vi "JUnit Full.vi"() -> ()   [LabVIEW 2013]
doc: "This example illustrates how to create a complete JUnit XML report."
uses:
  JUnit XML/Test Suites/Test Suites.lvclass
  <vilib>/xml/Close Reference(Node).vi
  <vilib>/xml/NI_XML.lvlib
  <resource>/objmgr/DOMUserDefRef.rc
  JUnit XML/Test Case/Test Case.lvclass
  JUnit XML/Test Suite/Test Suite.lvclass
  JUnit XML/Property/Property.lvclass
panel:
  out "XML":string
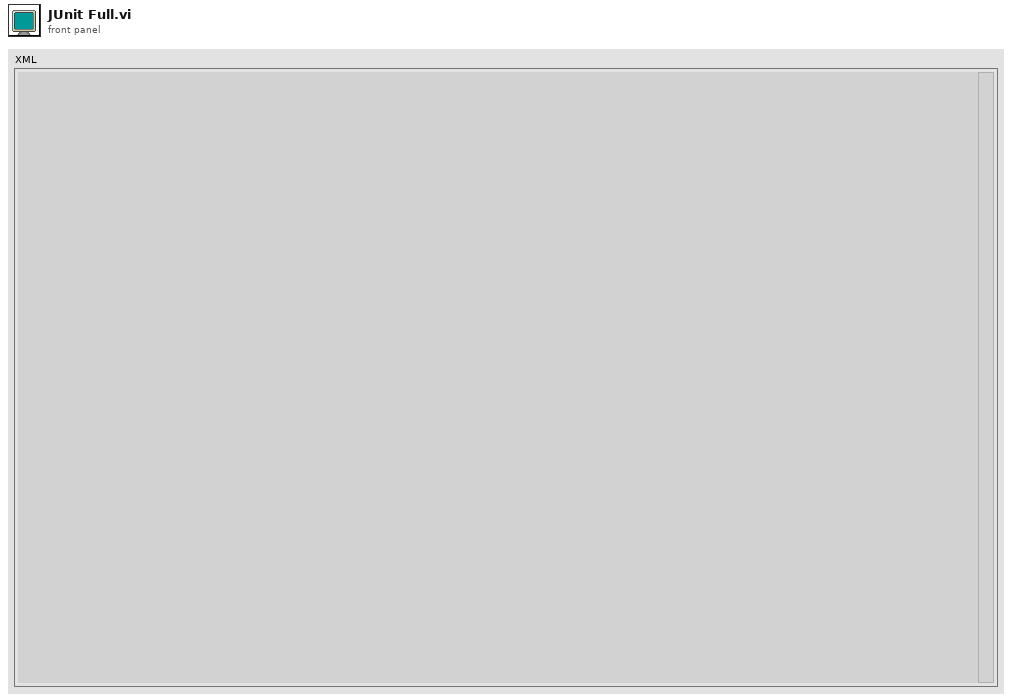
[diagram p1: front panel]
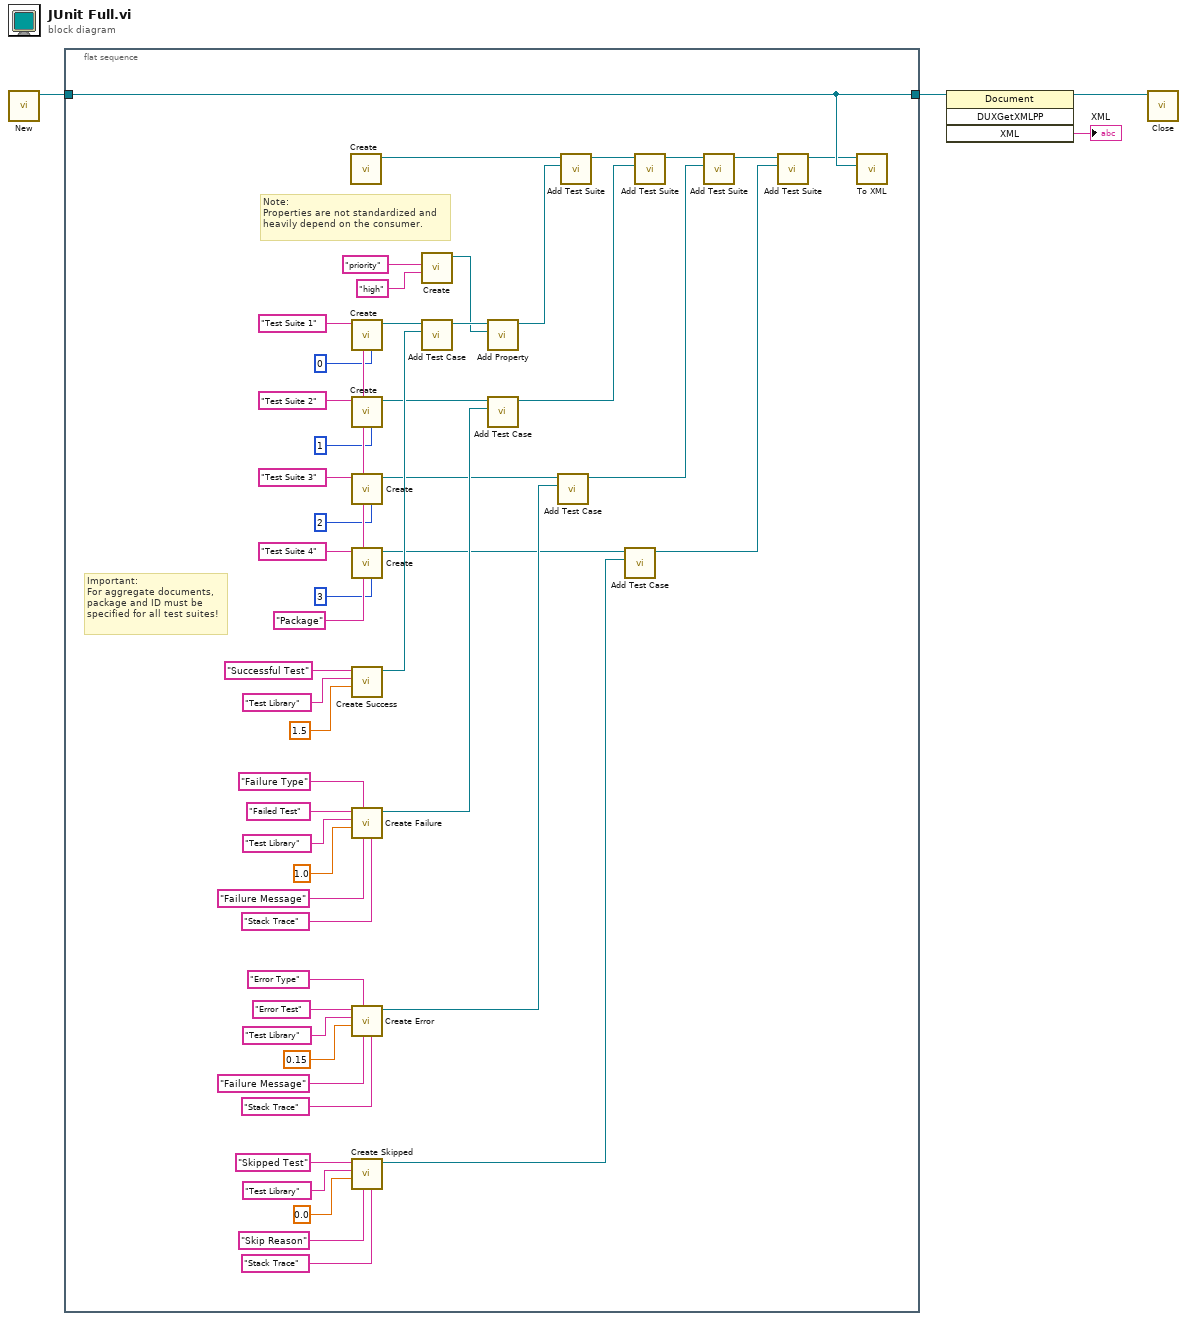
[diagram p0: block diagram]
diagram:
  n1 = call <vilib>:"New.vi"() -> ("DOM document out"=w4:refnum<k20>)  [unwired: 8 in, 1 out]
  n2 = flat-sequence {
    tunnel: w4 -> [w49]
    tunnel: [w49] -> w2
    frame #0 {
      w14 = "Package" ("Package (\"\" = undefined)")
      # "Note:\nProperties are not standardized and\nheavily depend on the consumer."
      # "Important:\nFor aggregate documents,\npackage and ID must be\nspecified for all test suites!"
      n3 = call "Create.vi"() -> ("Test Suites"=w28:refnum<class "Test Suites.lvclass">)  [unwired: 10 in, 1 out]
      n4 = call "Create.vi"("Id (-1 = undefined)"=0, "Package (\"\" = undefined)"=w14, "Name"="Test Suite 1") -> ("Test Suite"=w51:refnum<class "Test Suite.lvclass">)  [unwired: 7 in, 1 out]
      n5 = call "Create.vi"("Id (-1 = undefined)"=1, "Package (\"\" = undefined)"=w14, "Name"="Test Suite 2") -> ("Test Suite"=w24:refnum<class "Test Suite.lvclass">)  [unwired: 7 in, 1 out]
      n6 = call "Create.vi"("Id (-1 = undefined)"=2, "Package (\"\" = undefined)"=w14, "Name"="Test Suite 3") -> ("Test Suite"=w23:refnum<class "Test Suite.lvclass">)  [unwired: 7 in, 1 out]
      n7 = call "Create.vi"("Id (-1 = undefined)"=3, "Package (\"\" = undefined)"=w14, "Name"="Test Suite 4") -> ("Test Suite"=w22:refnum<class "Test Suite.lvclass">)  [unwired: 7 in, 1 out]
      n8 = call "Create Success.vi"("Time"=1.5, "Classname"="Test Library", "Name"="Successful Test") -> ("Test Case"=w50:refnum<class "Test Case.lvclass">)  [unwired: 7 in, 1 out]
      n9 = call "Create Failure.vi"("Stack Trace"="Stack Trace", "Message"="Failure Message", "Type"="Failure Type", "Time"=1.0, "Classname"="Test Library", "Name"="Failed Test") -> ("Test Case"=w42:refnum<class "Test Case.lvclass">)  [unwired: 4 in, 1 out]
      n10 = call "Create Error.vi"("Stack Trace"="Stack Trace", "Message"="Failure Message", "Type"="Error Type", "Time"=0.15, "Classname"="Test Library", "Name"="Error Test") -> ("Test Case"=w35:refnum<class "Test Case.lvclass">)  [unwired: 4 in, 1 out]
      n11 = call "Create Skipped.vi"("Stack Trace"="Stack Trace", "Message"="Skip Reason", "Time"=0.0, "Classname"="Test Library", "Name"="Skipped Test") -> ("Test Case"=w29:refnum<class "Test Case.lvclass">)  [unwired: 5 in, 1 out]
      n12 = call "Create.vi"("Value"="high", "Name"="priority") -> ("Property"=w7:refnum<class "Property.lvclass">)  [unwired: 8 in, 1 out]
      n13 = call "Add Test Case.vi"("Test Case"=w50, "Test Suite in"=w51) -> ("Test Suite out"=w9:refnum<class "Test Suite.lvclass">)  [unwired: 8 in, 1 out]
      n14 = call "Add Property.vi"("Property"=w7, "Test Suite in"=w9) -> ("Test Suite out"=w8:refnum<class "Test Suite.lvclass">)  [unwired: 8 in, 1 out]
      n15 = call "Add Test Case.vi"("Test Case"=w42, "Test Suite in"=w24) -> ("Test Suite out"=w20:refnum<class "Test Suite.lvclass">)  [unwired: 8 in, 1 out]
      n16 = call "Add Test Case.vi"("Test Case"=w35, "Test Suite in"=w23) -> ("Test Suite out"=w19:refnum<class "Test Suite.lvclass">)  [unwired: 8 in, 1 out]
      n17 = call "Add Test Suite.vi"("Test Suite"=w8, "Test Suites in"=w28) -> ("Test Suites out"=w21:refnum<class "Test Suites.lvclass">)  [unwired: 8 in, 1 out]
      n18 = call "Add Test Case.vi"("Test Case"=w29, "Test Suite in"=w22) -> ("Test Suite out"=w17:refnum<class "Test Suite.lvclass">)  [unwired: 8 in, 1 out]
      n19 = call "Add Test Suite.vi"("Test Suite"=w20, "Test Suites in"=w21) -> ("Test Suites out"=w18:refnum<class "Test Suites.lvclass">)  [unwired: 8 in, 1 out]
      n20 = call "Add Test Suite.vi"("Test Suite"=w19, "Test Suites in"=w18) -> ("Test Suites out"=w16:refnum<class "Test Suites.lvclass">)  [unwired: 8 in, 1 out]
      n21 = call "Add Test Suite.vi"("Test Suite"=w17, "Test Suites in"=w16) -> ("Test Suites out"=w15:refnum<class "Test Suites.lvclass">)  [unwired: 8 in, 1 out]
      n22 = call-dynamic "To XML.vi"("Parent"=w49, "Test Suites in"=w15) -> ()  [unwired: 9 in, 1 out]
    }
  }
  n23 = invoke class="Document" method="DUXGetXMLPP"(reference=w2) -> (reference out=w3:refnum<k20>, "XML"=→"XML":string)  [unwired: 3 in, 2 out]
  n24 = call-poly <vilib>:"Close.vi"("node"=w3) -> ()  [unwired: 8 in, 1 out]
